vi "读软件版本（授权用）.vi"(9 "CAN端口":u16(ring) items=["0", "1"], 10 "设备索引号":u16(ring) items=["0", "1", "2", "3", "4", "5", "6", "7", "8", "9", "10", "11", "12", "13", "14", "15", ""], 11 "CAN卡类型":u32(ring)=4 items=["PCI5121"=1, "PCI9810"=2, "USBCAN1"=3, "USBCAN2"=4, "PCI9820"=5, "PCI5110"=7, "CANLite(mini)"=8, "ISA9620"=9, "ISA5420"=10, "PC104CAN"=11, "DNP9810"=13, "PCI9840B"=14, "PC104C2"=15, "PCI9820I"=16, "pec9920"=18, "USBCAN_E_U"=20, "USBCAN_2E_U"=21]) -> (0 "编号":string, 3 "项目软件版本":string)   [LabVIEW 2013]
panel:
  out "布尔":bool=TRUE
  in  "VCI_Receive":T1 {"Rsv3" max=0 format="%x"; "Rsv2" min=101 format="%x"; "Rsv1" format="%x"; "Data8" format="%x"; "Data7" format="%x"; "Data6" format="%x"; "Data5" format="%x"; "Data4" format="%x"; "Data3" format="%x"; "Data2" format="%x"; "Data1" format="%x"; "DataLen" format="%x"; "ExternFlag" format="%x"; "RemoteFlag" format="%x"; "SendType" format="%x"; "TimeFlag" format="%x"; "TimeStamp" format="%x"; "ID" format="%x"}
  out "命令序号":u8
  in  "命令":u8 format="%x"
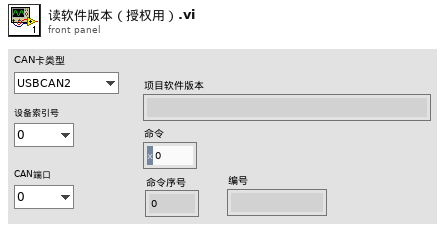
[diagram p1: front panel]
types:
  T1 = cluster{"ID":u32, "TimeStamp":u32, "TimeFlag":u8, "SendType":u8, "RemoteFlag":u8, "ExternFlag":u8, "DataLen":u8, "Data1":u8, "Data2":u8, "Data3":u8, "Data4":u8, "Data5":u8, "Data6":u8, "Data7":u8, "Data8":u8, "Rsv1":u8, "Rsv2":u8, "Rsv3":u8}
  T2 = cluster{"return type":u32, "pReceive":cluster{"ID":u32, "TimeStamp":u32, "TimeFlag":u8, "SendType":u8, "RemoteFlag":u8, "ExternFlag":u8, "DataLen":u8, "1":u8, "2":u8, "3":u8, "4":u8, "5":u8, "6":u8, "7":u8, "8":u8, "9":u8, "10":u8, "11":u8}[]}
  T3 = cluster{"ID":u32, "TimeStamp":u32, "TimeFlag":u8, "SendType":u8, "RemoteFlag":u8, "ExternFlag":u8, "DataLen":u8, "1":u8, "2":u8, "3":u8, "4":u8, "5":u8, "6":u8, "7":u8, "8":u8, "9":u8, "10":u8, "11":u8}[]
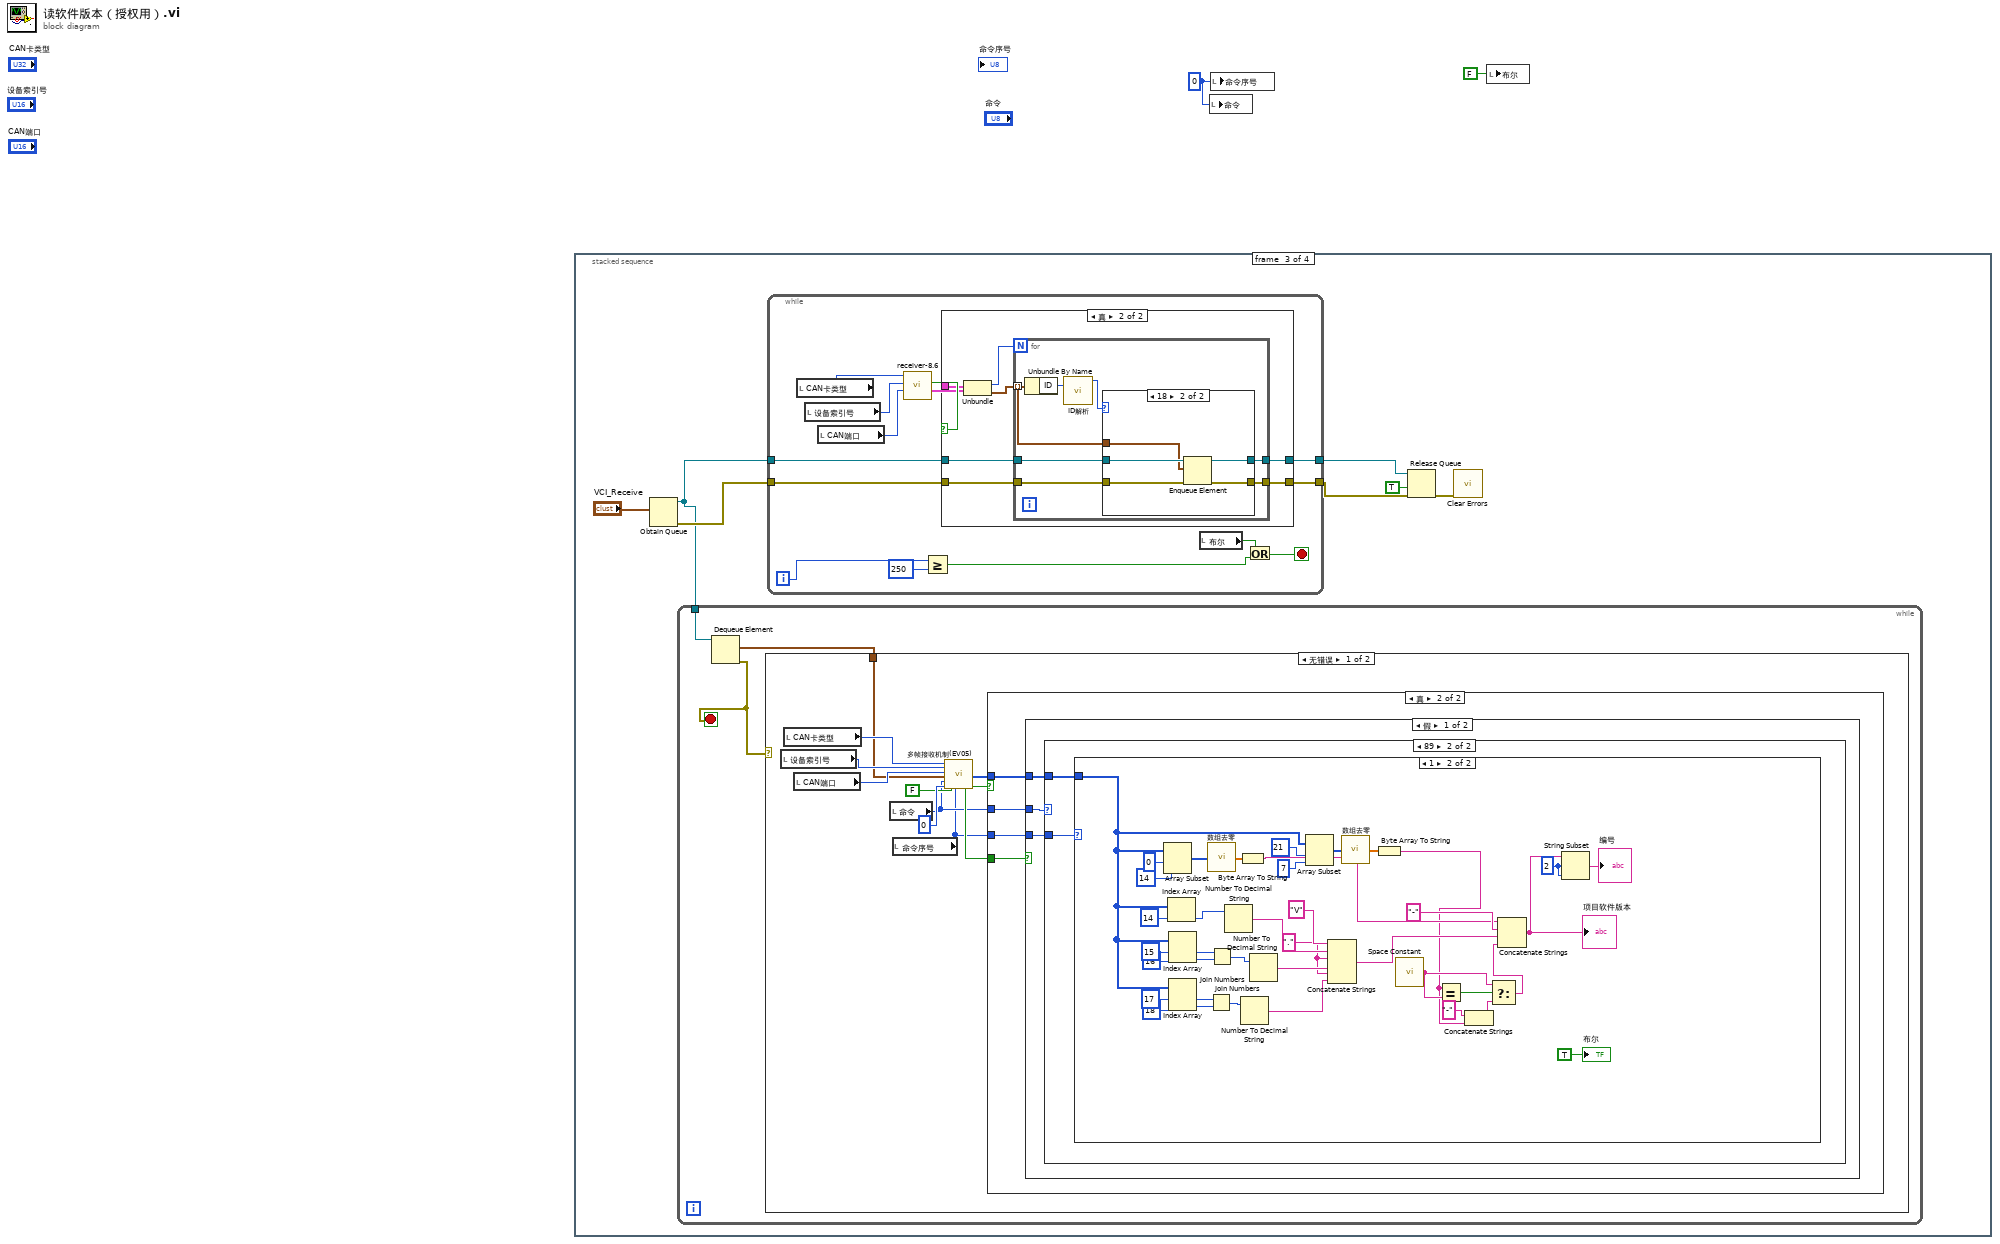
[diagram p0: block diagram]
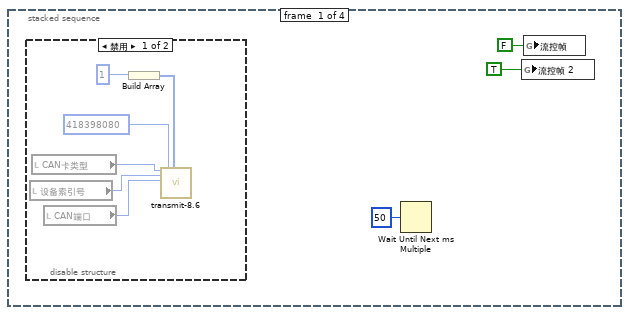
[diagram p2: hidden frame]
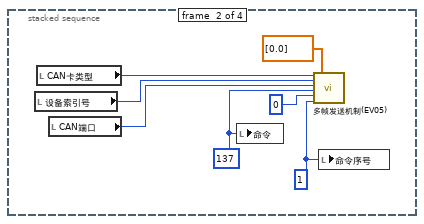
[diagram p4: hidden frame]
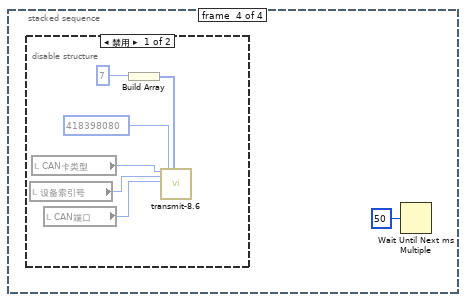
[diagram p12: hidden frame]
diagram:
  w2 = u8 0 ("命令序号")
  n1 = stacked-sequence {
    frame #0 {
      n2 = disable-structure shown="禁用" {
        frame Disabled {
          n3 = local read "设备索引号"() -> (w10:u16)
          n4 = local read "CAN卡类型"() -> (w11:u32)
          n5 = local read "CAN端口"() -> (w9:u16)
          n6 = Build Array(1) -> (w6:i32[])
          n7 = call "transmit-8.6.vi"("can卡类型"=w11, "设备索引号"=w10, "CAN端口"=w9, "ID"=418398080, "Data"=w6) -> ()  [unwired: 4 in, 11 out]
        }
        frame Enabled {
        }
      }
      n8 = Wait Until Next ms Multiple(millisecond multiple=u32 50 ("毫秒倍数")) -> ()  [unwired: 1 out]
      n9 = global write "EV05全局变量1.vi" "流控帧 2"(TRUE ("流控帧 2")) -> ()
      n10 = global write "EV05全局变量1.vi" "流控帧"(FALSE ("流控帧")) -> ()
    }
    frame #1 {
      w13 = u32 1 ("命令序号")
      w15 = u8 137 ("命令")
      n11 = local read "设备索引号"() -> (w17:u16)
      n12 = local read "CAN卡类型"() -> (w18:u32)
      n13 = local read "CAN端口"() -> (w16:u16)
      n14 = local write "命令"(w15) -> ()
      n15 = call "多帧发送机制(EV05).vi"("can卡类型"=w18, "设备索引号"=w17, "CAN端口"=w16, "命令"=w15, "板号"=u8 0, "命令序号"=w13, "输入数据"=dbl[] [0.0]) -> ()  [unwired: 1 in, 12 out]
      n16 = local write "命令序号"(w13) -> ()
    }
    frame #2 {
      n17 = Obtain Queue(element data type="VCI_Receive") -> (queue out=w20:refnum<queue>, error out=w24:errorcluster)  [unwired: 4 in, 1 out]
      n18 = while {
        tunnel: w20 -> [w28]
        stop <- w26 stop-if-true
        n19 = Dequeue Element(queue=w28) -> (element=w27:T1, error out=w26:errorcluster)  [unwired: 2 in, 2 out]
        n20 = case shown="无错误" w26 {
          tunnel: w27 -> [w36 _]
          frame No Error {
            n21 = local read "设备索引号"() -> (w38:u16)
            n22 = local read "CAN卡类型"() -> (w39:u32)
            n23 = local read "CAN端口"() -> (w37:u16)
            n24 = local read "命令"() -> (w31:u8)
            n25 = local read "命令序号"() -> (w30:u8)
            n26 = call "多帧接收机制(EV05).vi"("can卡类型"=w39, "设备索引号"=w38, "CAN端口"=w37, "VCI_Receive"=w36, "命令"=w31, "板号"=u32 0, "写?"=FALSE, "命令序号"=w30) -> ("错误信号"=w32:bool, "输出数组"=w29:u8[], "结束信号"=w33:bool)  [unwired: 9 out]
            n27 = case shown="真" w33 {
              tunnel: w32 -> [_ w43]
              tunnel: w31 -> [_ w42]
              tunnel: w30 -> [_ w41]
              tunnel: w29 -> [_ w40]
              frame False {
              }
              frame True {
                n28 = case shown="假" w43 {
                  tunnel: w42 -> [w46 _]
                  tunnel: w41 -> [w45 _]
                  tunnel: w40 -> [w44 _]
                  frame False {
                    n29 = case shown="89" w46 {
                      tunnel: w45 -> [_ w48]
                      tunnel: w44 -> [_ w47]
                      frame 0, Default {
                      }
                      frame 137 {
                        n30 = case shown="1" w48 {
                          tunnel: w47 -> [_ w53]
                          frame 0, Default {
                          }
                          frame 1 {
                            w50 = 2 ("偏移量(0)")
                            w58 = "." ("字符串")
                            n31 = Array Subset(array=w53, index=0 ("索引"), length=14 ("长度")) -> (w85:u8[])
                            n32 = Index Array(array=w53, index=14 ("索引")) -> (element=w75:u8)
                            n33 = Index Array(array=w53, index #1=15 ("索引"), index #2=16 ("索引")) -> (element #1=w81:u8, element #2=w82:u8)
                            n34 = Index Array(array=w53, index #1=17 ("索引"), index #2=18 ("索引")) -> (element #1=w76:u8, element #2=w77:u8)
                            n35 = call "数组去零.vi"("输入"=w85) -> ("输出"=w64:dbl[])
                            n36 = Join Numbers(hi=w76, lo=w77) -> ((hi.lo)=w73:u16)
                            n37 = Join Numbers(hi=w81, lo=w82) -> ((hi.lo)=w74:u16)
                            n38 = Number To Decimal String(number=w75) -> (decimal integer string=w68:string)  [unwired: 1 out]
                            n39 = Byte Array To String(unsigned byte array=w64) -> (string=w63:string)
                            n40 = Number To Decimal String(number=w73) -> (decimal integer string=w59:string)  [unwired: 1 out]
                            n41 = Number To Decimal String(number=w74) -> (decimal integer string=w67:string)  [unwired: 1 out]
                            n42 = Array Subset(array=w53, index=21 ("索引"), length=7 ("长度")) -> (w70:u8[])
                            n43 = Concatenate Strings("V" ("字符串"), w68, w58, w67, w58, w59) -> (w65:string)
                            n44 = call "数组去零.vi"("输入"=w70) -> ("输出"=w56:dbl[])
                            n45 = Byte Array To String(unsigned byte array=w56) -> (string=w54:string)
                            n46 = call <vilib>:"Space Constant.vi"() -> ("String"=w55:string)
                            n47 = Equal?(x=w54, y=w55) -> (x = y?=w60:bool)
                            n48 = Concatenate Strings("-" ("字符串"), w54) -> (w61:string)
                            n49 = Select(t=w55, s=w60, f=w61) -> (s? t:f=w57:string)
                            n50 = Concatenate Strings(w63, "-" ("字符串"), w65, w57) -> (w51:string)
                            "项目软件版本" <- w51
                            n51 = String Subset(string=w51, offset (0)=w50, length (rest)=w50) -> (substring=→"编号":string)
                            "布尔" <- TRUE
                          }
                        }
                      }
                    }
                  }
                  frame True {
                  }
                }
              }
            }
          }
          frame Error {
          }
        }
      }
      n52 = while {
        tunnel: w20 -> [w97]
        tunnel: w24 -> [w96]
        tunnel: [w95] -> w23
        tunnel: [w94] -> w22
        i -> [w93]
        stop <- w89 stop-if-true
        n53 = local read "CAN卡类型"() -> (w101:u32)
        n54 = local read "设备索引号"() -> (w100:u16)
        n55 = local read "CAN端口"() -> (w99:u16)
        n56 = call "receiver-8.6.vi"("CAN端口"=w99, "设备索引号"=w100, "CAN卡类型"=w101) -> ("输出簇"=w88:T2, "接收成功"=w98:bool)  [unwired: 1 in, 4 out]
        n57 = Greater Or Equal?(x=w93, y=250) -> (x >= y?=w90:bool)
        n58 = case shown="真" w98 {
          tunnel: w88 -> [_ w106]
          tunnel: w97 -> [w103 w110]
          tunnel: w96 -> [w102 w109]
          tunnel: [w103 w108] -> w95
          tunnel: [w102 w107] -> w94
          frame False {
          }
          frame True {
            n59 = Unbundle(w106) -> ("return type"=w105:u32, "pReceive"=w104:T3)
            n60 = for {
              N: w105 -> [_]
              tunnel: w110 -> [w115]
              tunnel: w109 -> [w114]
              tunnel: [w113] -> w108
              tunnel: [w112] -> w107
              tunnel: w104 -> [w111] mode=indexing
              n61 = Unbundle By Name(w111) -> ("ID"=w117:u32)
              n62 = call "ID解析.vi"("ID"=w117) -> ("PDU(1)"=w116:i32)  [unwired: 10 out]
              n63 = case shown="18" w116 {
                tunnel: w115 -> [w119 w124]
                tunnel: w114 -> [w118 w123]
                tunnel: [w119 w122] -> w113
                tunnel: [w118 w121] -> w112
                tunnel: w111 -> [_ w120]
                frame 0, Default {
                }
                frame 24 {
                  n64 = Enqueue Element(queue=w124, element=w120, error in (no error)=w123) -> (queue out=w122:refnum<queue>, error out=w121:errorcluster)  [unwired: 1 in, 1 out]
                }
              }
            }
          }
        }
        n65 = local read "布尔"() -> (w91:bool)
        n66 = Or(x=w91, y=w90) -> (x .or. y?=w89:bool)
      }
      n67 = Release Queue(queue=w23, force destroy? (F)=TRUE ("强制销毁？(F)"), error in (no error)=w22) -> (error out=w19:errorcluster)  [unwired: 2 out]
      n68 = call <vilib>:"Clear Errors.vi"("error in (no error)"=w19) -> ()  [unwired: 6 in, 1 out]
    }
    frame #3 {
      n69 = disable-structure shown="禁用" {
        frame Disabled {
          n70 = local read "设备索引号"() -> (w130:u16)
          n71 = local read "CAN卡类型"() -> (w131:u32)
          n72 = local read "CAN端口"() -> (w129:u16)
          n73 = Build Array(7) -> (w126:i32[])
          n74 = call "transmit-8.6.vi"("can卡类型"=w131, "设备索引号"=w130, "CAN端口"=w129, "ID"=418398080, "Data"=w126) -> ()  [unwired: 4 in, 11 out]
        }
        frame Enabled {
        }
      }
      n75 = Wait Until Next ms Multiple(millisecond multiple=u32 50 ("毫秒倍数")) -> ()  [unwired: 1 out]
    }
  }
  n76 = local write "命令"(w2) -> ()
  n77 = local write "命令序号"(w2) -> ()
  n78 = local write "布尔"(FALSE ("布尔")) -> ()
